vi "ReadData_5160_only.vi"(10 "Buffer mode":T1, 11 "scope params":T2={"scope mode"=enum."Stopped", "ticker"=refnum, "5160 samples per trigger"=0, "FPGA ref"=refnum, "P2P params"={"instrument handle"="", "stream session"=refnum, "scale"={"offset"=0.0, "gain"=0.0, "reserved 1"=0.0, "reserved 2"=0.0}, "actual sample rate"=10000000.0, "Trigger"=enum."PFI 0", "SCOPE Resource"="Dev1", "input impedance"=0}, "data mode"=enum."Real IO", "5782 samples per record"=0, "Chart length"=0, "RemoteConnection"=refnum, "last phase"=[]} {"P2P params"."input impedance" items=["1 mega ohm"=0, "50 ohms"=2]; "P2P params"."actual sample rate" format="%.2p"}) -> (1 "Num elements":i32, 2 "data":dbl[][](array[numeric]) format="%.2f", 3 "scope params out":T2={"scope mode"=enum."Stopped", "ticker"=refnum, "5160 samples per trigger"=0, "FPGA ref"=refnum, "P2P params"={"instrument handle"="", "stream session"=refnum, "scale"={"offset"=0.0, "gain"=0.0, "reserved 1"=0.0, "reserved 2"=0.0}, "actual sample rate"=10000000.0, "Trigger"=enum."PFI 0", "SCOPE Resource"="Dev1", "input impedance"=0}, "data mode"=enum."Real IO", "5782 samples per record"=0, "Chart length"=0, "RemoteConnection"=refnum, "last phase"=[]} {"P2P params"."input impedance" items=["1 mega ohm"=0, "50 ohms"=2]; "P2P params"."actual sample rate" format="%.2p"})   [LabVIEW 2013]
uses:
  controls/scope_params.ctl
  Utilities/Ticker/Ticker.lvclass
  Communication/Driver/RemoteConnection/RemoteConnection.lvclass
  controls/ScopeMode.ctl
  Config/FPGAref.ctl
  P2P streaming/P2P params.ctl
  P2P streaming/trigger_source.ctl
  FPGA/DataMode.ctl
  controls/Data_display_mode.ctl
  <vilib>/rvi/interface/common/niFpgaWaitOnOcc.vi
  <vilib>/Utility/error.llb/Error Cluster From Error Code.vi
  <vilib>/rvi/errors/niLvFpgaAdjustHostInterfaceError.vi
  <vilib>/rvi/interface/nirviMethod/nirviMethod.xnode
  <vilib>/rvi/interface/nirviReadWriteControl/nirviReadWriteControl.xnode
  NiFpgaLv.dll
  <vilib>/rvi/interface/Simulation/niFpgaSimulationCallBeginRW.vi
  <vilib>/FPGAPlugInAG/Dynamic/niLvFpga_ReadFifo_Dynamic.vi
  <vilib>/rvi/errors/niLvFpgaMergeErrorWithErrorCode.vi
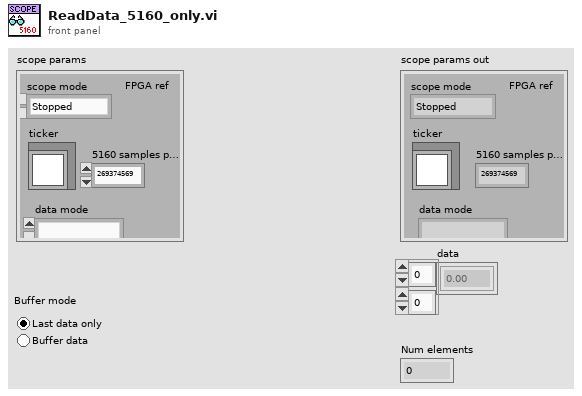
[diagram p1: front panel]
types:
  T1 = typedef "Data_display_mode.ctl" = enum32{"Last data only", "Buffer data"}
  T2 = typedef "scope_params.ctl" = cluster{"scope mode":T3, "ticker":refnum<class "Ticker.lvclass">, "5160 samples per trigger":u32, "FPGA ref":T4, "P2P params":T5, "data mode":T7, "5782 samples per record":u32, "Chart length":i32, "RemoteConnection":refnum<class "RemoteConnection.lvclass">, "last phase":dbl[]}
  T3 = typedef "ScopeMode.ctl" = enum16{"Stopped", "Single", "Running", "Continuous"}
  T4 = typedef "FPGAref.ctl" = refnum<k20>
  T5 = typedef "P2P params.ctl" = cluster{"instrument handle":refnum<k15>, "stream session":refnum<k20>, "scale":cluster{"offset":dbl, "gain":dbl, "reserved 1":dbl, "reserved 2":dbl}, "actual sample rate":dbl, "Trigger":T6, "SCOPE Resource":refnum<k15>, "input impedance":u32}
  T6 = typedef "trigger_source.ctl" = enum16{"PFI 0", "PFI 1", "Software"}
  T7 = typedef "DataMode.ctl" = enum16{"Real IO", "Simulated"}
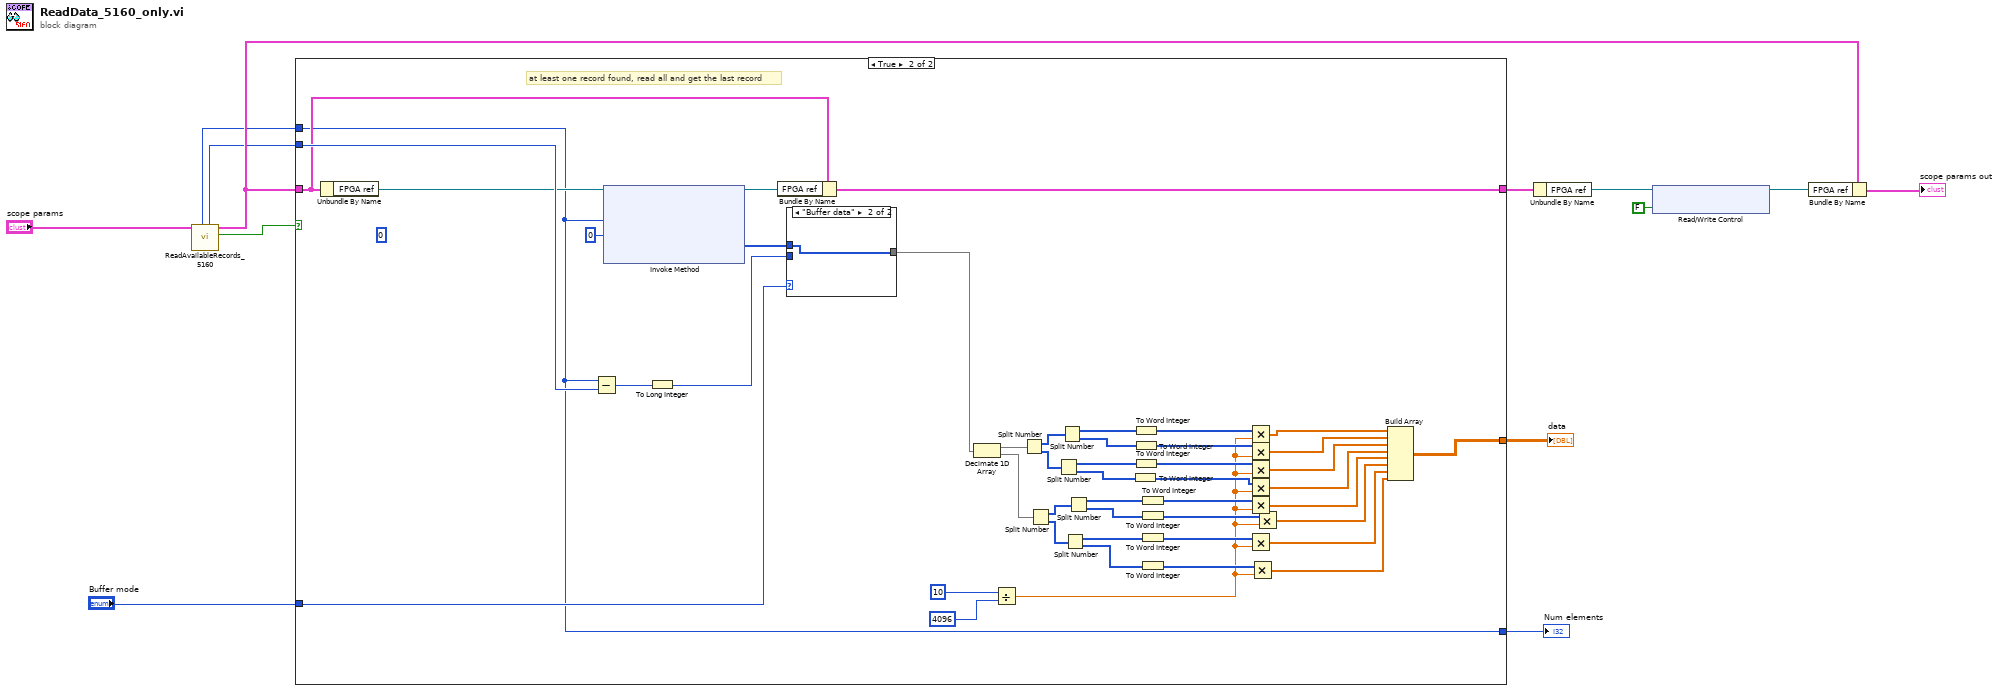
[diagram p0: block diagram]
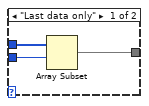
[diagram p3: hidden frame]
diagram:
  n1 = call "ReadAvailableRecords_5160.vi"("scope params"="scope params") -> ("record available"=w4:bool, "scope params out"=w7:T2, "last record size 5160"=w2:u32, "#elements 5160"=w1:u32)  [unwired: 7 in]
  n2 = case shown="True" w4 {
    tunnel: [_ w37] -> w13
    tunnel: [_ w15] -> w12
    tunnel: w7 -> [w14 w40]
    tunnel: [w14 w38] -> w6
    tunnel: w2 -> [_ w41]
    tunnel: w1 -> [_ w15]
    tunnel: "Buffer mode" -> [_ w42]
    frame False {
    }
    frame True {
      (unwired) 0 ("Timeout (ms)")
      # "at least one record found, read all and get the last record"
      n3 = Unbundle By Name(w40) -> ("FPGA ref"=w16:T4)
      n4 = Subtract(x=w15, y=w41) -> (x-y=w45:u32)
      n5 = xnode "Invoke Method"("FPGA VI Reference In"=w16, "Number of Elements"=w15, "Timeout (ms)"=0) -> ("FPGA VI Reference Out"=w39:T4, "Data"=w43:u64[])  [unwired: 1 in, 2 out]
      n6 = To Long Integer(number=w45) -> (32bit integer=w46:i32)
      n7 = Bundle By Name(cluster=w40, "FPGA ref"=w39) -> (w38:T2)
      n8 = case shown="\"Buffer data\"" w42 {
        tunnel: w43 -> [w63 w64]
        tunnel: w46 -> [w62 _]
        tunnel: [w61 w64] -> w36
        frame "Last data only" {
          n9 = Array Subset(array=w63, index=w62) -> (w61:u64[])  [unwired: 1 in]
        }
        frame "Buffer data" {
        }
      }
      n10 = Decimate 1D Array(w36) -> (w54:u64[], w47:u64[])
      n11 = Divide(x=10, y=4096) -> (x/y=w17:dbl)
      n12 = Split Number(x=w54) -> (hi(x)=w56:u32[], lo(x)=w60:u32[])
      n13 = Split Number(x=w47) -> (hi(x)=w52:u32[], lo(x)=w48:u32[])
      n14 = Split Number(x=w60) -> (hi(x)=w58:u16[], lo(x)=w57:u16[])
      n15 = Split Number(x=w56) -> (hi(x)=w55:u16[], lo(x)=w59:u16[])
      n16 = Split Number(x=w48) -> (hi(x)=w50:u16[], lo(x)=w51:u16[])
      n17 = Split Number(x=w52) -> (hi(x)=w53:u16[], lo(x)=w49:u16[])
      n18 = To Word Integer(number=w57) -> (16bit integer=w32:i16[])
      n19 = To Word Integer(number=w55) -> (16bit integer=w35:i16[])
      n20 = To Word Integer(number=w59) -> (16bit integer=w34:i16[])
      n21 = To Word Integer(number=w58) -> (16bit integer=w33:i16[])
      n22 = To Word Integer(number=w53) -> (16bit integer=w31:i16[])
      n23 = To Word Integer(number=w49) -> (16bit integer=w30:i16[])
      n24 = To Word Integer(number=w50) -> (16bit integer=w29:i16[])
      n25 = To Word Integer(number=w51) -> (16bit integer=w28:i16[])
      n26 = Multiply(x=w35, y=w17) -> (x*y=w27:dbl[])
      n27 = Multiply(x=w34, y=w17) -> (x*y=w26:dbl[])
      n28 = Multiply(x=w33, y=w17) -> (x*y=w25:dbl[])
      n29 = Multiply(x=w32, y=w17) -> (x*y=w24:dbl[])
      n30 = Multiply(x=w31, y=w17) -> (x*y=w23:dbl[])
      n31 = Multiply(x=w29, y=w17) -> (x*y=w21:dbl[])
      n32 = Multiply(x=w28, y=w17) -> (x*y=w20:dbl[])
      n33 = Multiply(x=w30, y=w17) -> (x*y=w22:dbl[])
      n34 = Build Array(w27, w26, w25, w24, w23, w22, w21, w20) -> (w37:dbl[][])
    }
  }
  "data" <- w13
  "Num elements" <- w12
  n35 = Unbundle By Name(w6) -> ("FPGA ref"=w5:T4)
  n36 = xnode "Read/Write Control"("FPGA VI Reference In"=w5, "Trigger simulated data"=FALSE) -> ("FPGA VI Reference Out"=w10:T4)  [unwired: 1 in, 1 out]
  n37 = Bundle By Name(cluster=w7, "FPGA ref"=w10) -> (→"scope params out":T2)
